vi "Read Identification String.vi"(8 "error in (no error)":errorcluster, 10 "node":u8, 11 "ProPar in":refnum<class "PL Bronkhorst ProPar.lvclass">) -> (0 "error out":errorcluster, 2 "id string":string, 3 "ProPar out":refnum<class "PL Bronkhorst ProPar.lvclass">)   [LabVIEW 2015, in "PL Bronkhorst ProPar.lvclass"]
doc: "Reads identification string of the specified <b>node</b>."
uses:
  PL Bronkhorst ProPar.lvclass
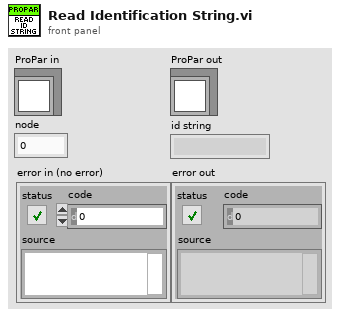
[diagram p1: front panel]
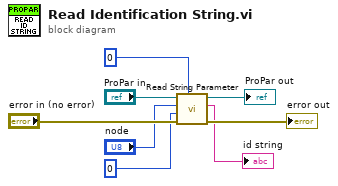
[diagram p0: block diagram]
diagram:
  n1 = call "Read String Parameter.vi"("process number"=u8 0, "error in (no error)"="error in (no error)", "parameter number"=u8 0 ("process number"), "node"="node", "ProPar in"="ProPar in") -> ("error out"=→"error out":errorcluster, "value"=→"id string":string, "ProPar out"=→"ProPar out":refnum<class "PL Bronkhorst ProPar.lvclass">)  [unwired: 4 in]
